vi "independent_strober.vi"(7 "light pulse (s)":dbl, 8 "error in (no error)":errorcluster, 9 "LED CHANNELS":dbl[](array[numeric]), 10 "LED_TABLE":dbl[][](array[numeric]), 11 "Iteration in":u32) -> (0 "error out":errorcluster, 3 "Iteration out":u32)   [LabVIEW 2013]
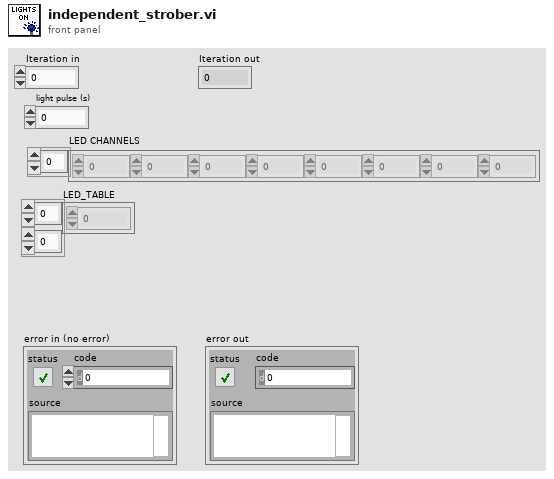
[diagram p1: front panel]
types:
  T1 = enum16{"Set Mode", "Set Normal Current ", "Set Strobe Parameters", "Set Normal Parameters", "Set Strobe Profile "}
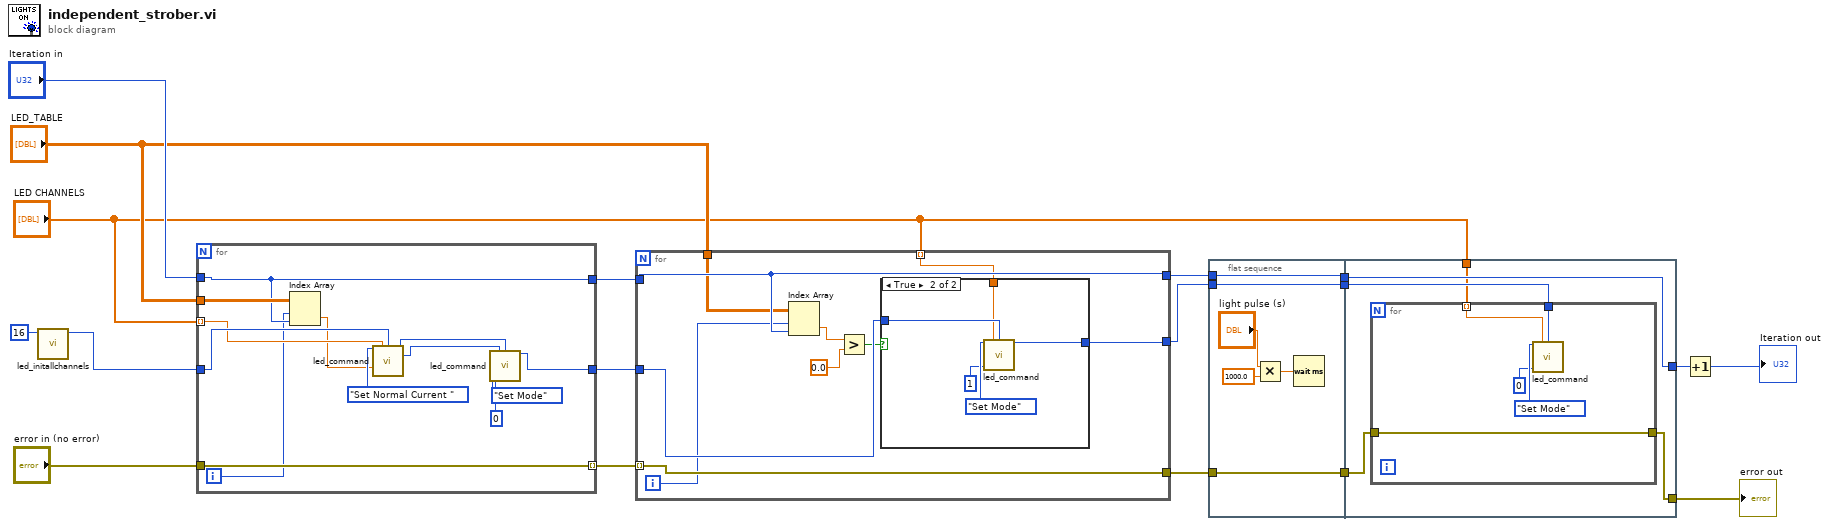
[diagram p0: block diagram]
diagram:
  n1 = call "led_initallchannels.vi"("Channels"=16) -> ("Device Handle Out"=w6:u32)  [unwired: 9 in, 1 out]
  n2 = for {
    tunnel: "error in (no error)" -> [w31]
    tunnel: [w31] -> w14 mode=indexing
    tunnel: w6 -> [w25]
    tunnel: [w24] -> w15
    tunnel: "LED_TABLE" -> [w23]
    tunnel: "LED CHANNELS" -> [w22] mode=indexing
    tunnel: "Iteration in" -> [w21]
    tunnel: [w21] -> w3
    i -> [w20]
    n3 = Index Array(array=w23, index (row)=w20, index (col)=w21) -> (element=w19:dbl)
    n4 = call "led_command.vi"("COMMAND"=T1."Set Normal Current ", "Channel"=w22, "Device Handle"=w25, "Iset"=w19) -> ("Device Handle Out"=w27:u32, "Channel Out"=w28:i32)  [unwired: 8 in, 2 out]
    n5 = call "led_command.vi"("COMMAND"=T1."Set Mode", "Channel"=w28, "Device Handle"=w27, "Mode"=u32 0) -> ("Device Handle Out"=w24:u32)  [unwired: 8 in, 3 out]
  }
  n6 = for {
    tunnel: w3 -> [w36]
    tunnel: w15 -> [w41]
    tunnel: [w40] -> w8
    tunnel: [w36] -> w9
    tunnel: [w39] -> w11
    tunnel: w14 -> [w39] mode=indexing
    tunnel: "LED_TABLE" -> [w35]
    tunnel: "LED CHANNELS" -> [w32] mode=indexing
    i -> [w34]
    n7 = Index Array(array=w35, index (row)=w34, index (col)=w36) -> (element=w33:dbl)
    n8 = Greater?(x=w33, y=0.0) -> (0:w37:bool)
    n9 = case shown="True" w37 {
      tunnel: w41 -> [w42 w45]
      tunnel: [w42 w44] -> w40
      tunnel: w32 -> [_ w43]
      frame False {
      }
      frame True {
        n10 = call "led_command.vi"("COMMAND"=T1."Set Mode", "Channel"=w43, "Device Handle"=w45, "Mode"=u32 1) -> ("Device Handle Out"=w44:u32)  [unwired: 8 in, 3 out]
      }
    }
  }
  n11 = flat-sequence {
    tunnel: w8 -> [w51]
    tunnel: [w51] -> w18
    tunnel: w9 -> [w50]
    tunnel: [w50] -> w17
    tunnel: w11 -> [w49]
    tunnel: [w49] -> w16
    tunnel: w18 -> [w58]
    tunnel: w17 -> [w57]
    tunnel: [w57] -> w10
    tunnel: w16 -> [w56]
    tunnel: [w55] -> w12
    tunnel: "LED CHANNELS" -> [w54]
    frame #0 {
      n12 = Multiply(x="light pulse (s)", y=1000.0) -> (x*y=w53:dbl)
      n13 = Wait (ms)(milliseconds to wait=w53) -> ()  [unwired: 1 out]
    }
    frame #1 {
      n14 = for {
        tunnel: w58 -> [w61]
        tunnel: w56 -> [w60]
        tunnel: [w60] -> w55
        tunnel: w54 -> [w59] mode=indexing
        n15 = call "led_command.vi"("COMMAND"=T1."Set Mode", "Channel"=w59, "Device Handle"=w61, "Mode"=u32 0) -> ()  [unwired: 8 in, 4 out]
      }
    }
  }
  n16 = Increment(x=w10) -> (x+1=→"Iteration out":u32)
  "error out" <- w12
